vi "Resolve Template Value.vi"(6 "Locals":refnum<class "Value Tree.lvclass">, 7 "Folder":path, 8 "error in (no error)":errorcluster, 9 "Template Service in":refnum<class "TemplateService.lvclass">, 10 "Variable Name":string, 11 "TemplateVariableResolver in":refnum<class "IncludeResolver.lvclass">) -> (0 "error out":errorcluster, 1 "Template Service":refnum<class "TemplateService.lvclass">, 2 "Value":refnum<class "Value Tree.lvclass">)   [LabVIEW 2023, in "HTTP Server.lvlib" / "IncludeResolver.lvclass"]
uses:
  IncludeResolver.lvclass
  IncludeResolver.lvclass/IncludeResolver.ctl
  TemplateService/TemplateService.lvclass
  Value Tree/Value Tree.lvclass
  HTTP Server.lvlib
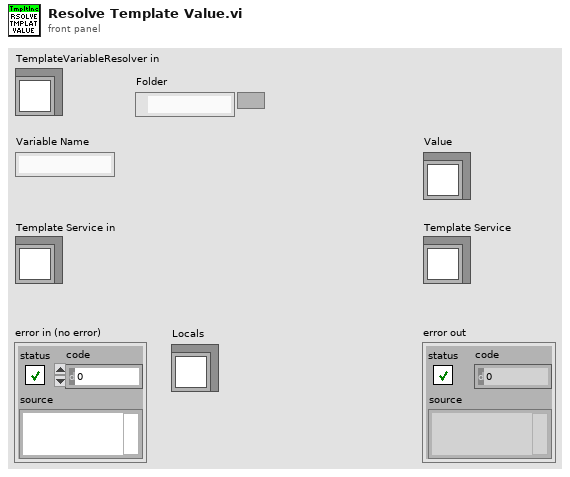
[diagram p1: front panel]
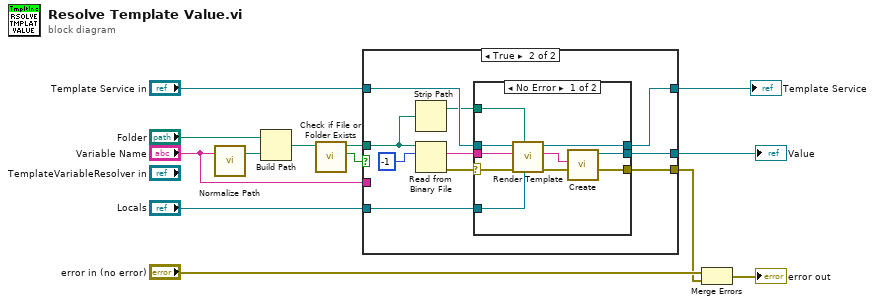
[diagram p0: block diagram]
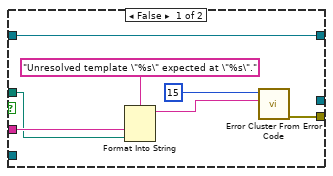
[diagram p2: hidden frame]
diagram:
  n1 = call "Normalize Path.vi"("Path String"="Variable Name") -> ("Path"=w11:path)  [unwired: 6 in]
  n2 = Build Path(base path="Folder", name or relative path=w11) -> (appended path=w5:path)
  n3 = call <vilib>:"Check if File or Folder Exists.vi"("path"=w5) -> ("file or folder exists?"=w10:bool, "dup path"=w9:path)  [unwired: 8 in, 1 out]
  n4 = case shown="True" w10 {
    tunnel: w9 -> [w14 w30]
    tunnel: [w20 w26] -> w8
    tunnel: "Template Service in" -> [w20 w25]
    tunnel: [w15 w23] -> w2
    tunnel: [_ w22] -> w6
    tunnel: "Variable Name" -> [w17 _]
    tunnel: "Locals" -> [_ w21]
    frame False {
      n5 = Format Into String(format string="Unresolved template \"%s\" expected at \"%s\".", w17, w14) -> (resulting string=w16:string)  [unwired: 2 in, 1 out]
      n6 = call <vilib>:"Error Cluster From Error Code.vi"("error message (\"\")"=w16, "error code (0)"=15) -> ("error out"=w15:errorcluster)  [unwired: 7 in]
    }
    frame True {
      n7 = Strip Path(path=w30) -> (stripped path=w24:path)  [unwired: 1 out]
      n8 = Read from Binary File(10:-1 ("count (1)"), 11:w30) -> (0:w27:errorcluster, 2:w29:string)  [unwired: 4 in, 2 out]
      n9 = case shown="No Error" w27 {
        selector: w27 -> [w37 w41]
        tunnel: w25 -> [w39 w40]
        tunnel: w29 -> [w38 _]
        tunnel: [w36 w41] -> w23
        tunnel: [w31 _] -> w22
        tunnel: w24 -> [w35 _]
        tunnel: [w34 w40] -> w26
        tunnel: w21 -> [w33 _]
        frame No Error {
          n10 = call-dynamic "Render Template.vi"("Locals (None)"=w33, "Folder"=w35, "error in (no error)"=w37, "Template"=w38, "TemplateService in"=w39) -> ("error out"=w36:errorcluster, "Output"=w32:string, "TemplateService out"=w34:refnum<class "TemplateService.lvclass">)  [unwired: 4 in]
          n11 = call "Create.vi"("Value"=w32) -> ("Value Tree out"=w31:refnum<class "Value Tree.lvclass">)  [unwired: 10 in]
        }
        frame Error {
        }
      }
    }
  }
  "Value" <- w6
  "Template Service" <- w8
  n12 = Merge Errors("error in (no error)", w2) -> (→"error out":errorcluster)
